vi "TESmart Test.vi"() -> ()   [LabVIEW 2020]
uses:
  <vilib>/Instr/_visa.llb/VISA Flush IO Buffer Mask.ctl
  563c3848-c783-4633-9a5f-64a6460e93d3.vi
  <vilib>/Instr/_visa.llb/VISA Configure Serial Port (Instr).vi
  TESmart Utils/TESmart Utils.lvlib
panel:
  out "Serial Settings:Number of Bytes at Serial Port":u32
  out "Routes":i32[](array[numeric])
  out "error out":errorcluster
  out "read buffer":string
  in  "VISA resource name":refnum<visa-resource-name>
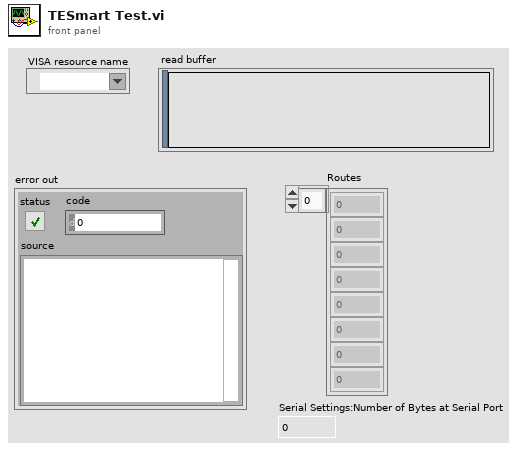
[diagram p1: front panel]
types:
  T1 = typedef "VISA Flush IO Buffer Mask.ctl" = u16
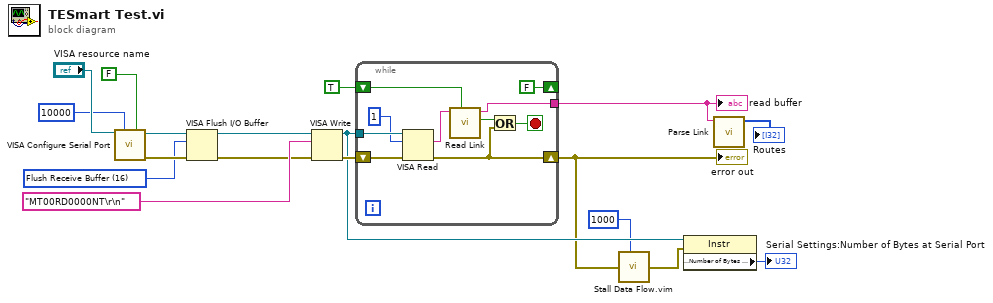
[diagram p0: block diagram]
diagram:
  w6 = T1 16 items=["Flush Receive Buffer"=16, "Write Transmit Buffer to Device"=32, "Flush Receive Buffer (No I/O)"=64, "Flush Transmit Buffer"=128] ("Mask")
  n1 = call-poly "VISA Configure Serial Port"("VISA resource name"="VISA resource name", "timeout (10sec)"=u32 10000, "Enable Termination\nChar (T)"=FALSE ("Enable Termination\nChar (T)")) -> ("VISA resource name out"=w9:refnum<visa-resource-name>, "error out"=w10:errorcluster)  [unwired: 11 in]
  n2 = VISA Flush I/O Buffer(VISA resource name=w9, mask (16)=w6, error in (no error)=w10) -> (VISA resource name out=w8:refnum<visa-resource-name>, error out=w7:errorcluster)
  n3 = VISA Write(VISA resource name=w8, write buffer="MT00RD0000NT\r\n", error in (no error)=w7) -> (VISA resource name out=w5:refnum<visa-resource-name>, error out=w14:errorcluster)  [unwired: 1 out]
  n4 = while {
    tunnel: w5 -> [w27]
    shift-right: [w21] -> w3
    shift-left: w14 -> [w28]
    shift-right: [FALSE] -> _
    shift-left: TRUE -> [w24]
    tunnel: [w19] -> w12
    stop <- w20 stop-if-true
    n5 = VISA Read(VISA resource name=w27, byte count=u32 1, error in (no error)=w28) -> (read buffer=w25:string, error out=w21:errorcluster)  [unwired: 2 out]
    n6 = call "Read Link.vi"("Reset? (F)"=w24, "Input"=w25) -> ("End?"=w22:bool, "Full Output"=w19:string)  [unwired: 8 in]
    n7 = Or(x=w22, y=w21) -> (x .or. y?=w20:bool)
  }
  "read buffer" <- w12
  "error out" <- w3
  n8 = call "Stall Data Flow.vim"("value in"=w3, "milliseconds to wait"=u32 1000) -> ("value out"=w2:errorcluster)  [unwired: 1 out]
  n9 = property class="Instr"(reference=w5, error in=w2) -> ("Serial Settings:Number of Bytes at Serial Port"=→"Serial Settings:Number of Bytes at Serial Port":u32)  [unwired: 2 out]
  n10 = call "Parse Link.vi"("String"=w12) -> ("Routes"=→"Routes":i32[])  [unwired: 10 in]
